vi "Arry2XYdata.vi"(6 "ClusterSigFormat":T2, 8 "MporofSelSgs":refnum<vi>, 9 "Value":T1, 10 "ArrySelectedSig":refnum<vi>, 11 "Array输入":refnum<vi>) -> (3 "数组":cluster{"时间(s)":dbl[], "数据":dbl[]}[](array[cluster]))   [LabVIEW 2015]
uses:
  Ctrls/YesOrNo.ctl
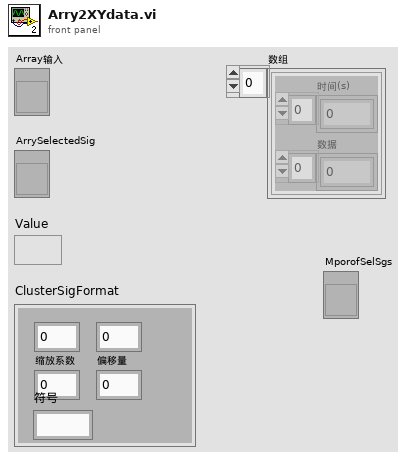
[diagram p1: front panel]
types:
  T1 = typedef "YesOrNo.ctl" = bool
  T2 = cluster{"起始位":u8, "长度":u8, "缩放系数":dbl, "偏移量":dbl, "符号":string}
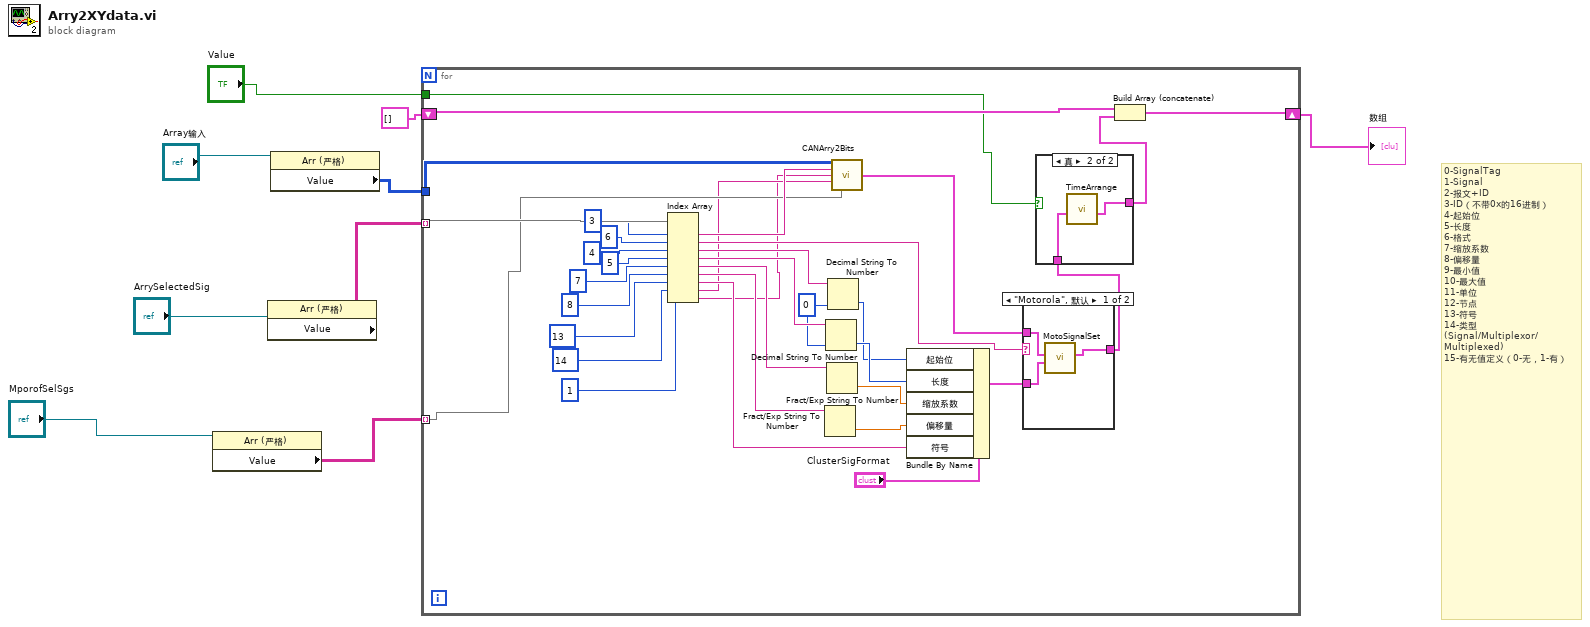
[diagram p0: block diagram]
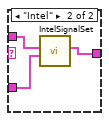
[diagram p3: hidden frame]
diagram:
  # "0-SignalTag\n1-Signal\n2-报文+ID\n3-ID（不带0x的16进制）\n4-起始位\n5-长度\n6-格式\n7-缩放系数\n8-偏移量\n9-最小值\n10-最大值\n11-单位\n12-节点\n13-符号\n14-类型\n(Signal/Multiplexor/\nMultiplexed)\n15-有无值定义（0-无，1-有）"
  n1 = property class="Arr (严格)"(reference="MporofSelSgs") -> ("Value"=w1:string[][])  [unwired: 1 in, 2 out]
  n2 = property class="Arr (严格)"(reference="ArrySelectedSig") -> ("Value"=w5:string[][])  [unwired: 1 in, 2 out]
  n3 = property class="Arr (严格)"(reference="Array输入") -> ("Value"=w7:u32[][])  [unwired: 1 in, 2 out]
  n4 = for {
    tunnel: w7 -> [w28]
    tunnel: w5 -> [w43] mode=indexing
    shift-right: [w30] -> w3
    shift-left: cluster{"时间(s)":dbl[], "数据":dbl[]}[] [] -> [w29]
    tunnel: "Value" -> [w15]
    tunnel: w1 -> [w13] mode=indexing
    w31 = u8 0 ("默认(0 I32)")
    n5 = Index Array(array=w43, index #1=3 ("索引"), index #2=6 ("索引"), index #3=4 ("索引"), index #4=5 ("索引"), index #5=7 ("索引"), index #6=8 ("索引"), index #7=13 ("索引"), index #8=14 ("索引"), index #9=1 ("索引")) -> (element #1=w41:string, element #2=w40:string, element #3=w33:string, element #4=w32:string, element #5=w26:string, element #6=w27:string, element #7=w23:string, element #8=w12:string, element #9=w10:string)
    n6 = Fract/Exp String To Number(string=w27) -> (number=w22:dbl)  [unwired: 3 in, 1 out]
    n7 = Decimal String To Number(string=w32, default (0L)=w31) -> (number=w20:u8)  [unwired: 1 in, 1 out]
    n8 = Fract/Exp String To Number(string=w26) -> (number=w21:dbl)  [unwired: 3 in, 1 out]
    n9 = Decimal String To Number(string=w33, default (0L)=w31) -> (number=w19:u8)  [unwired: 1 in, 1 out]
    n10 = call "CANArry2Bits.vi"("重构的Data数组输入"=w28, "CAN_ID"=w41, "Signal"=w10, "Style"=w12, "mpor"=w13) -> ("CAN64B簇"=w39:cluster{"时间(s)":dbl[], "Data64Bits(u64)":u64[]})  [unwired: 8 in, 2 out]
    n11 = Bundle By Name(cluster="ClusterSigFormat", "起始位"=w19, "长度"=w20, "缩放系数"=w21, "偏移量"=w22, "符号"=w23) -> (w18:T2)
    n12 = case shown="\"Motorola\", 默认" w40 {
      tunnel: w39 -> [w49 w52]
      tunnel: w18 -> [w48 w51]
      tunnel: [w47 w50] -> w17
      frame "Motorola", Default {
        n13 = call "MotoSignalSet.vi"("CAN64B簇"=w49, "信号格式簇"=w48) -> ("信号"=w47:cluster{"时间(s)":dbl[], "数据":dbl[]})  [unwired: 6 in]
      }
      frame "Intel" {
        n14 = call "IntelSignalSet.vi"("CAN64B簇"=w52, "信号格式簇"=w51) -> ("信号"=w50:cluster{"时间(s)":dbl[], "数据":dbl[]})  [unwired: 6 in]
      }
    }
    n15 = case shown="真" w15 {
      tunnel: w17 -> [w44 w46]
      tunnel: [w44 w45] -> w16
      frame False {
      }
      frame True {
        n16 = call "TimeArrange.vi"("Din"=w46) -> ("Dout"=w45:cluster{"时间(s)":dbl[], "数据":dbl[]})  [unwired: 9 in]
      }
    }
    n17 = Build Array (concatenate)(w29, w16) -> (w30:cluster{"时间(s)":dbl[], "数据":dbl[]}[])
  }
  "数组" <- w3
